vi "HEWH Force Terminate Condition During Last Draw.vi"(6 "HEWH Specific DAQ":T1, 9 "Current Sequence Index":i32, 10 "Terminate Condition in":T5, 11 "PRAT/RLT Sequence":T6[](array[typedef]) {"Time" format="%<%H:%M:%S>t"}) -> (3 "Terminate Condition out":T5)   [LabVIEW 2019]
uses:
  Type Definitions/PRAT Test.ctl
  Utility/Save File/File Setup (Public)/Type Definition/Save File HEWH Heating Control Mode.ctl
  Draw Water Specific/Type Definitions/Terminate Draw Conditions.ctl
  Type Definitions/HEWH Start Conditions.ctl
  Draw Water Specific/Type Definitions/Check Special Condtions.ctl
  Draw Water Specific/Type Definitions/HEWH Special Condition Check.ctl
  Type Definitions/HEWH Draw Flag ENUM.ctl
  Type Definitions/HEWH Specific DAQ.ctl
  Type Definitions/HEWH Power Data.ctl
  Type Definitions/HEWH Power Elements.ctl
  Utility/Type Definitions/UTILITY Power Analyzer.ctl
  Utility/Save File/File Setup.lvlib
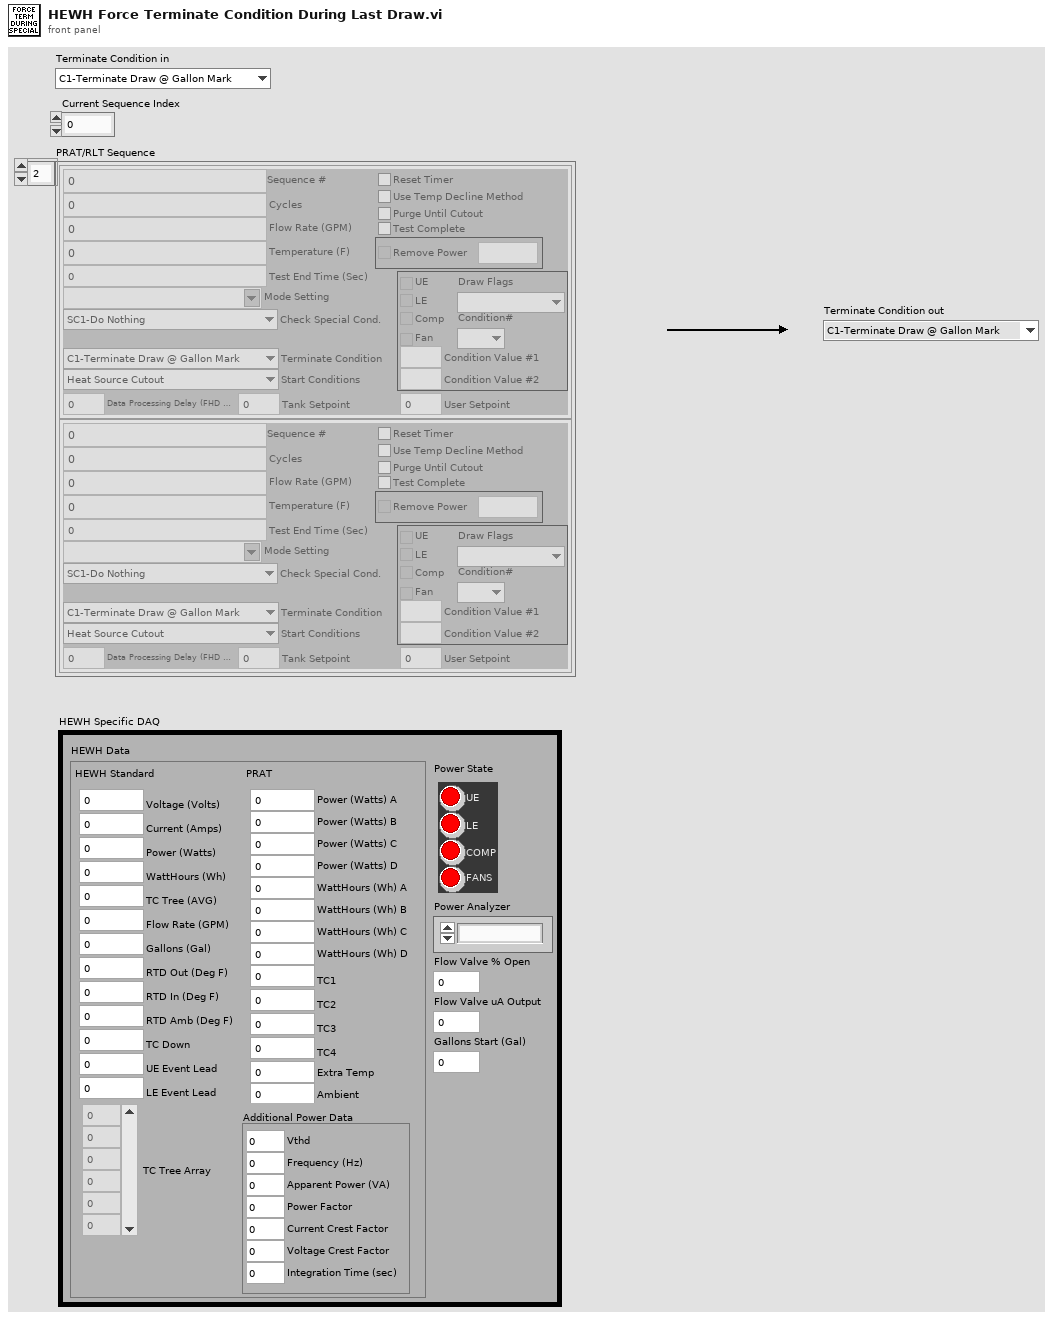
[diagram p1: front panel]
types:
  T1 = typedef "HEWH Specific DAQ.ctl" = cluster{"HEWH Data":T2, "Flow Valve % Open":dbl, "Power State":T3, "Power Analyzer":T4, "Flow Valve uA Output":i32, "Gallons Start (Gal)":dbl}
  T2 = typedef "HEWH Power Data.ctl" = cluster{"HEWH Standard":cluster{"Voltage (Volts)":dbl, "Current (Amps)":dbl, "Power (Watts)":dbl, "WattHours (Wh)":dbl, "TC Tree (AVG)":dbl, "Flow Rate (GPM)":dbl, "Gallons (Gal)":dbl, "RTD Out (Deg F)":dbl, "RTD In (Deg F)":dbl, "RTD Amb (Deg F)":dbl, "TC Down":dbl, "UE Event Lead":i32, "LE Event Lead":i32, "TC Tree Array":dbl[]}, "PRAT":cluster{"Power (Watts) A":dbl, "Power (Watts) B":dbl, "Power (Watts) C":dbl, "Power (Watts) D":dbl, "TC1":dbl, "TC2":dbl, "TC3":dbl, "TC4":dbl, "WattHours (Wh) A":dbl, "WattHours (Wh) B":dbl, "WattHours (Wh) C":dbl, "WattHours (Wh) D":dbl, "Ambient":dbl, "Extra Temp":dbl}, "Additional Power Data":cluster{"Vthd":dbl, "Frequency (Hz)":dbl, "Apparent Power (VA)":dbl, "Power Factor":dbl, "Current Crest Factor":dbl, "Voltage Crest Factor":dbl, "Integration Time (sec)":dbl}}
  T3 = typedef "HEWH Power Elements.ctl" = cluster{"UE":bool, "LE":bool, "COMP":bool, "FANS":bool}
  T4 = typedef "UTILITY Power Analyzer.ctl" = enum16{"", "APLUS", "WT210", "WT500", "WT300", "OSI", "Debug", "WT230", "WT300_1", "WT300_2"}
  T5 = typedef "Terminate Draw Conditions.ctl" = enum16{"C1-Terminate Draw @ Gallon Mark", "C2-Special Last Draw (HU Test)", "C3-RTD Out <=", "C4-Mean Tank Temp <=", "C5-Decrease RTD Out (Deg F)", "C6-Time (Seconds)", "C7-Until Any Heat Source", "C8-Specific Heat Source", "C9-Do Nothing", "C10-Inlet Outlet RTD Temp Delta"}
  T6 = typedef "PRAT Test.ctl" = cluster{"Sequence #":dbl, "Cycles":i32, "Mode Setting":T7, "Flow Rate (GPM)":dbl, "Temperature (F)":dbl, "Reset Timer":bool, "Use Temp Decline Method":bool, "Terminate Condition":T5, "Condition Value #1":dbl, "UE":bool, "LE":bool, "Comp":bool, "Fan":bool, "Test End Time (Sec)":dbl, "Purge Until Cutout":bool, "Start Conditions":T8, "Condition Value #2":dbl, "Remove Power":bool, "Time":dbl, "Check Special Cond.":T9, "Condition#":T10, "Draw Flags":T11, "Data Processing Delay (FHD 15sec, UEF 5 Sec)":dbl, "Test Complete":bool, "User Setpoint":dbl, "Tank Setpoint":dbl}
  T7 = typedef "File Setup.lvlib/Save File HEWH Heating Control Mode.ctl" = string
  T8 = typedef "HEWH Start Conditions.ctl" = enum16{"Heat Source Cutout", "At Time (Seconds)", "Every X (Seconds)", "T2 >= X° Below Setpoint", "Seconds From Complete", "Wait for LE & Comp Cutout", "Wait for Comp Cutout", "Wait for LE Cutout", "Wait for UE Cutout", "Start Immediately"}
  T9 = typedef "Check Special Condtions.ctl" = enum16{"SC1-Do Nothing", "SC2-Check Heat Source (On-C2/Off-C1)", "SC3-Check Skip Condition", "SC4-Check Heat Source ON/Fail", "SC5-Keep Draw Valves Open", "SC6-Skip Purge"}
  T10 = typedef "HEWH Special Condition Check.ctl" = enum16{"N/A", "C1", "C2", "Reset/Fail", "Skip Draw Sequence"}
  T11 = typedef "HEWH Draw Flag ENUM.ctl" = enum16{"N/A", "None(0)", "Sml(1)", "Med(2)", "SmlMed(3)", "Lrg(4)", "SmlLrg(5)", "MedLrg(6)", "SmlMedLrg(7)"}
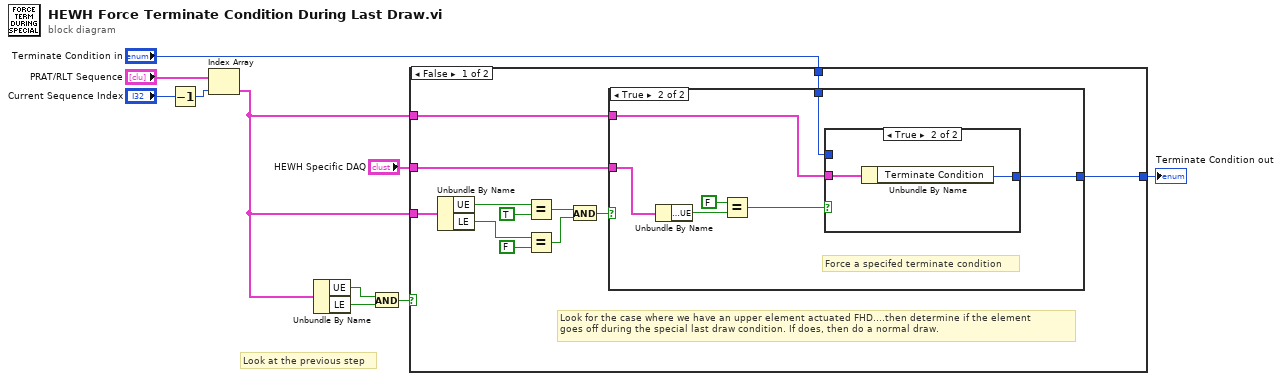
[diagram p0: block diagram]
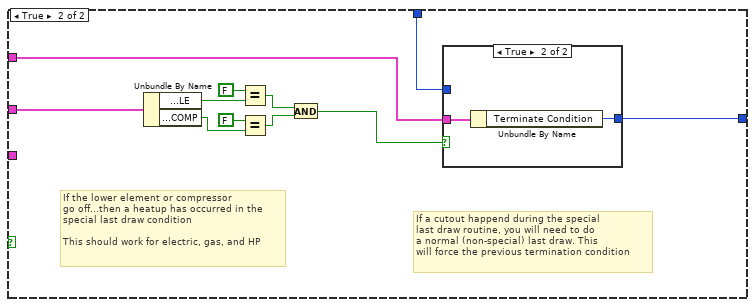
[diagram p4: hidden frame]
diagram:
  # "Look at the previous step"
  n1 = Decrement(x="Current Sequence Index") -> (x-1=w9:i32)
  n2 = Index Array(array="PRAT/RLT Sequence", index=w9) -> (element=w4:T6)
  n3 = Unbundle By Name(w4) -> ("UE"=w6:bool, "LE"=w5:bool)
  n4 = And(x=w6, y=w5) -> (x .and. y?=w1:bool)
  n5 = case shown="False" w1 {
    tunnel: "HEWH Specific DAQ" -> [w22 w44]
    tunnel: w4 -> [w21 _]
    tunnel: w4 -> [w13 w43]
    tunnel: "Terminate Condition in" -> [w12 w42]
    tunnel: [w11 w41] -> w2
    frame False {
      # "Look for the case where we have an upper element actuated FHD....then determine if the element \ngoes off during the special last draw condition. If does, then do a normal draw."
      n6 = Unbundle By Name(w21) -> ("UE"=w20:bool, "LE"=w17:bool)
      n7 = Equal?(x=w20, y=TRUE) -> (x = y?=w16:bool)
      n8 = Equal?(x=w17, y=FALSE) -> (x = y?=w15:bool)
      n9 = And(x=w16, y=w15) -> (x .and. y?=w14:bool)
      n10 = case shown="True" w14 {
        tunnel: w22 -> [_ w30]
        tunnel: w13 -> [_ w26]
        tunnel: w12 -> [w23 w27]
        tunnel: [w23 w24] -> w11
        frame False {
        }
        frame True {
          # "Force a specifed terminate condition"
          n11 = Unbundle By Name(w30) -> ("Power State.UE"=w25:bool)
          n12 = Equal?(x=FALSE, y=w25) -> (x = y?=w29:bool)
          n13 = case shown="True" w29 {
            tunnel: w27 -> [w31 _]
            tunnel: [w31 w33] -> w24
            tunnel: w26 -> [_ w32]
            frame False {
            }
            frame True {
              n14 = Unbundle By Name(w32) -> ("Terminate Condition"=w33:T5)
            }
          }
        }
      }
    }
    frame True {
      # "If the lower element or compressor \ngo off...then a heatup has occurred in the \nspecial last draw condition\n\nThis should work for electric, gas, and HP"
      # "If a cutout happend during the special\nlast draw routine, you will need to do\na normal (non-special) last draw. This \nwill force the previous termination condition"
      n15 = Unbundle By Name(w44) -> ("Power State.LE"=w40:bool, "Power State.COMP"=w37:bool)
      n16 = Equal?(x=FALSE ("y"), y=w40) -> (x = y?=w36:bool)
      n17 = Equal?(x=FALSE ("y"), y=w37) -> (x = y?=w35:bool)
      n18 = And(x=w36, y=w35) -> (x .and. y?=w34:bool)
      n19 = case shown="True" w34 {
        tunnel: w42 -> [w45 _]
        tunnel: [w45 w47] -> w41
        tunnel: w43 -> [_ w46]
        frame False {
        }
        frame True {
          n20 = Unbundle By Name(w46) -> ("Terminate Condition"=w47:T5)
        }
      }
    }
  }
  "Terminate Condition out" <- w2
